vi "try_Web Browser Front Panel Control.vi"() -> ()   [LabVIEW 2026]
panel:
  out "Web Browser Control":string(html)="https://www.google.com/"
  in  "URL String":string
  in  "Stop":bool
  in  "Stop Load":bool
  in  "Reload":bool
  in  "Forward":bool
  in  "Back":bool
  # "Web Browser Control Demo"
  # "Instructions:\n1. Run the VI.\n2. Enter a URL String like \"www.ni.com\" or \"www.google.com\".\n3. Click links on the page, and use the Back, Forward, and Reload buttons to navigate pages.\n4. Click Stop to stop the VI, and close the VI when you are done with the demo. You do not need to save the VI."
  # "Close this VI when you are done with the demo."
  # "You do not need to save changes to this VI."
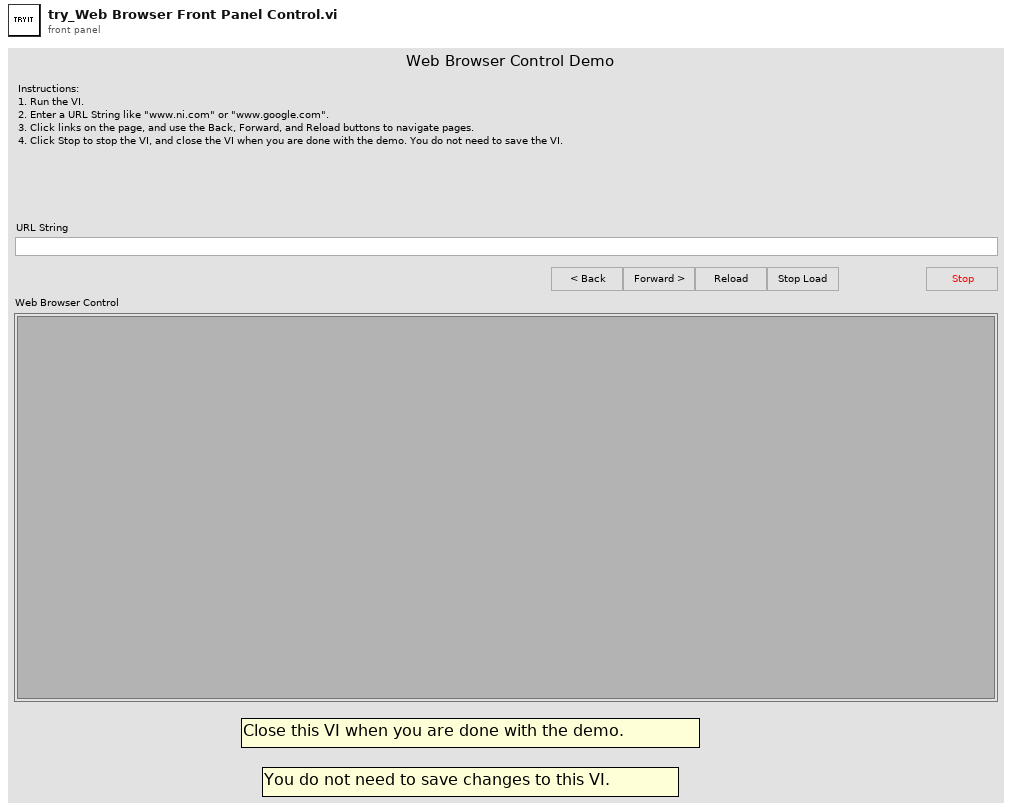
[diagram p1: front panel]
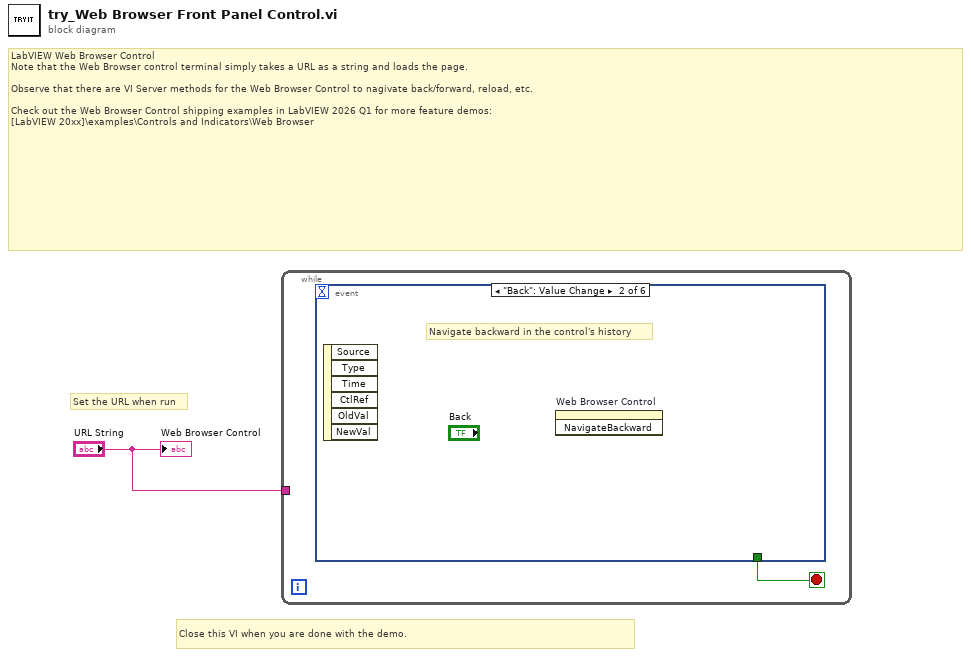
[diagram p0: block diagram]
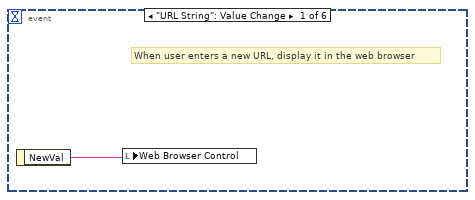
[diagram p2: hidden frame]
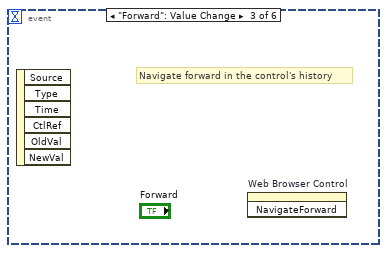
[diagram p3: hidden frame]
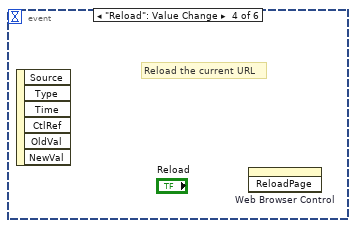
[diagram p4: hidden frame]
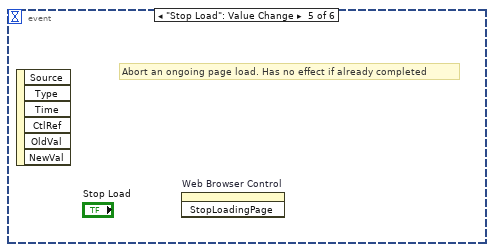
[diagram p5: hidden frame]
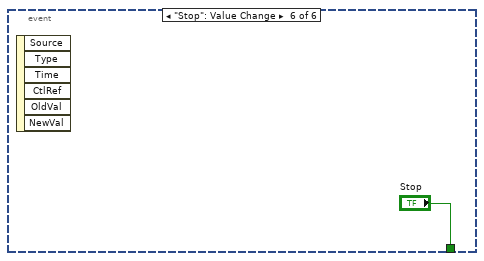
[diagram p6: hidden frame]
diagram:
  # "Set the URL when run"
  # "Close this VI when you are done with the demo."
  # "LabVIEW Web Browser Control\nNote that the Web Browser control terminal simply takes a URL as a string and loads the page.\n\nObserve that there are VI Server methods for the Web Browser Control to nagivate back/forward, reload, etc.\n\nCheck out the Web Browser Control shipping examples in LabVIEW 2026 Q1 for more feature demos:\n[LabVIEW 20xx]\\examples\\Controls and Indicators\\Web Browser"
  n1 = while {
    tunnel: "URL String" -> [_]
    stop <- w2 stop-if-true
    n2 = event shown="[1] \"Back\": Value Change" {
      selector: _ -> [_ _ _ _ _ _]
      dyn-events: _ -> [_ _ _ _ _ _]
      timeout: _ -> [_ _ _ _ _ _]
      tunnel: [_ _ _ _ _ "Stop"] -> w2
      event "URL String": Value Change {
        # "When user enters a new URL, display it in the web browser"
        n3 = event-data() -> ("NewVal"=w3:string)  [unwired: 1 in]
        n4 = local write "Web Browser Control"(w3) -> ()
      }
      event "Back": Value Change {
        # "Navigate backward in the control's history"
        n5 = event-data() -> ()  [unwired: 1 in, 6 out]
        n6 = invoke on="Web Browser Control" class="WebBrowser (strict)" method="NavigateBackward"() -> ()  [unwired: 3 in, 3 out]
      }
      event "Forward": Value Change {
        # "Navigate forward in the control's history"
        n7 = event-data() -> ()  [unwired: 1 in, 6 out]
        n8 = invoke on="Web Browser Control" class="WebBrowser (strict)" method="NavigateForward"() -> ()  [unwired: 3 in, 3 out]
      }
      event "Reload": Value Change {
        # "Reload the current URL"
        n9 = event-data() -> ()  [unwired: 1 in, 6 out]
        n10 = invoke on="Web Browser Control" class="WebBrowser (strict)" method="ReloadPage"() -> ()  [unwired: 3 in, 3 out]
      }
      event "Stop Load": Value Change {
        # "Abort an ongoing page load. Has no effect if already completed"
        n11 = event-data() -> ()  [unwired: 1 in, 6 out]
        n12 = invoke on="Web Browser Control" class="WebBrowser (strict)" method="StopLoadingPage"() -> ()  [unwired: 3 in, 3 out]
      }
      event "Stop": Value Change {
        n13 = event-data() -> ()  [unwired: 1 in, 6 out]
      }
    }
  }
  "Web Browser Control" <- "URL String"
